vi "correction for PL spectra.vi"(1 "file path (dialog if empty) 2":path caption="PL file needed to be transfromed") -> (0 "数组 2":dbl[][](array[numeric]))   [LabVIEW 2018]
uses:
  <vilib>/Utility/file.llb/Read Delimited Spreadsheet (DBL).vi
panel:
  out "first row":dbl[](array[numeric])
  out "XY Graph":cluster{"Y":dbl[], "Y":dbl[]}[](graph) caption="XY图"
  out "大小":i32
  out "数组":i32[](array[numeric])
  out "all rows 2":dbl[][](array[numeric]) caption="所有行"
  out "all rows":dbl[][](array[numeric]) caption="所有行"
  in  "file path (dialog if empty)":path=path "C:/PLQY corrected 20210803/correction file from 300nm to 1300nm 20230203.dat" caption="correction file from 300nm to 1300nm"
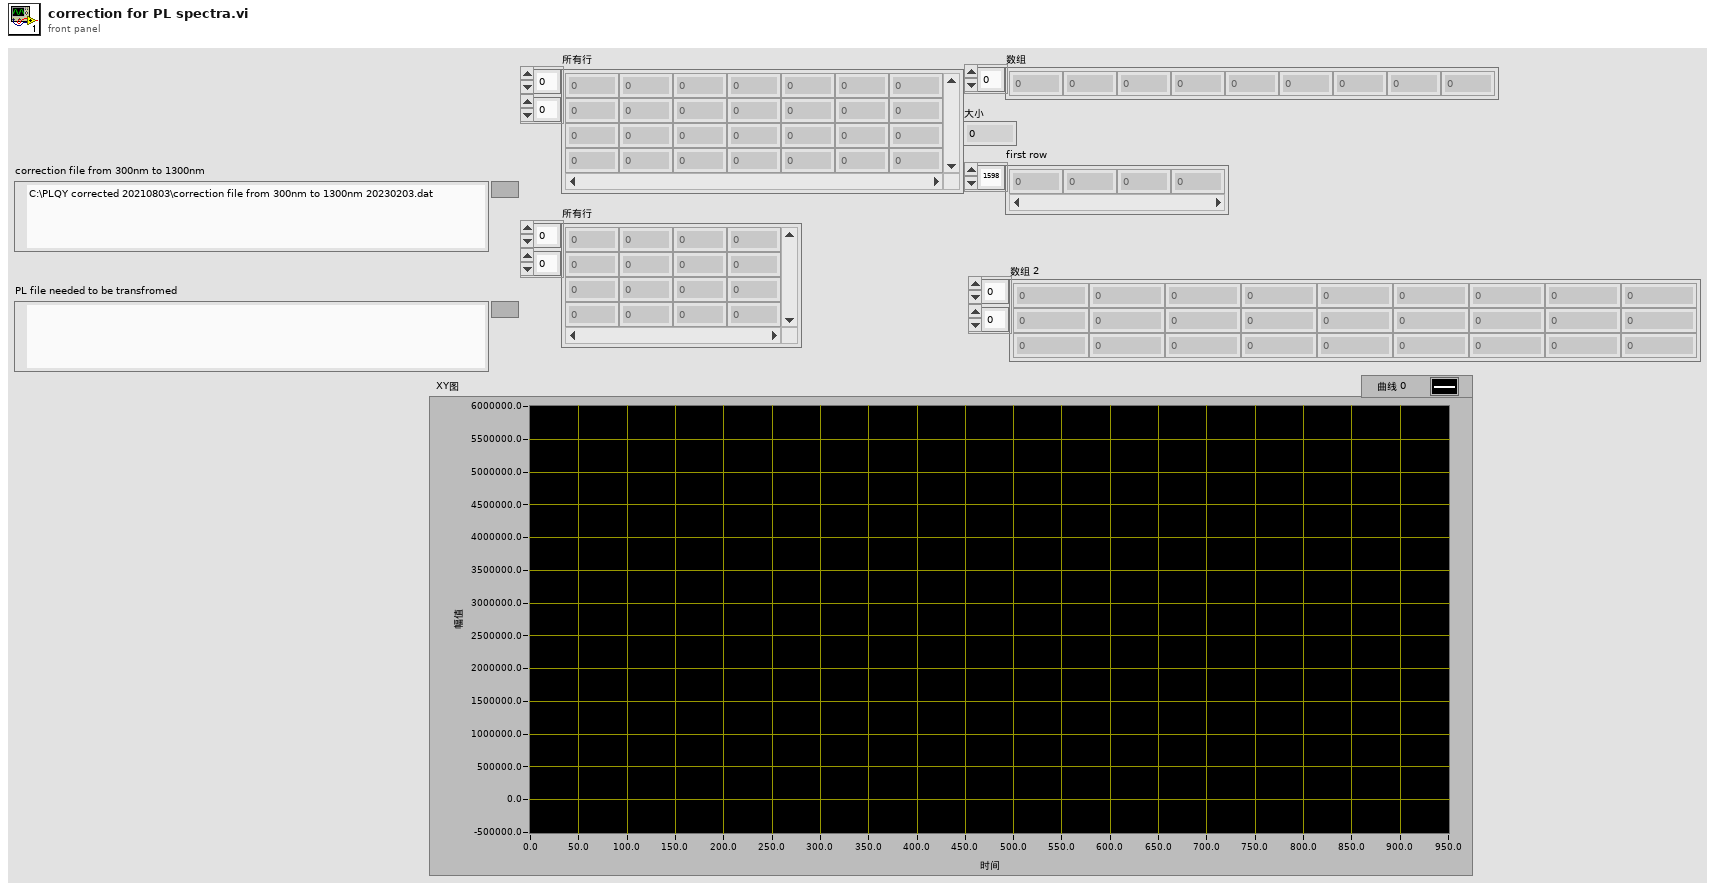
[diagram p1: front panel]
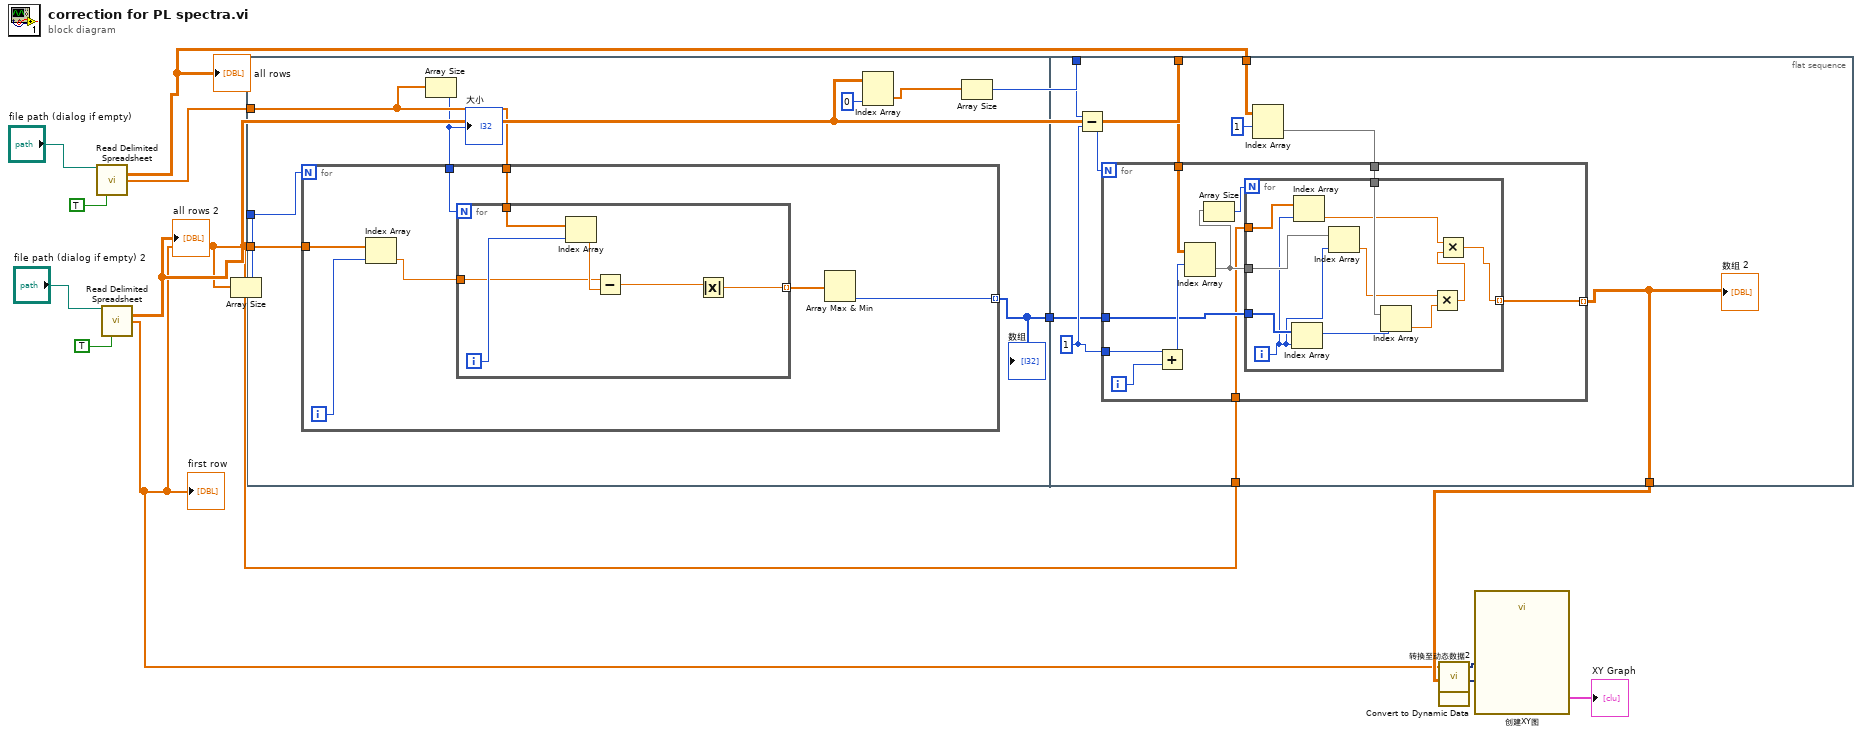
[diagram p0: block diagram]
diagram:
  n1 = call-poly <vilib>:"Read Delimited Spreadsheet.vi"("file path (dialog if empty)"="file path (dialog if empty)", "transpose? (F)"=TRUE) -> ("all rows"=w6:dbl[][], "first row"=w12:dbl[])  [unwired: 8 in, 4 out]
  "all rows" <- w6
  n2 = call-poly <vilib>:"Read Delimited Spreadsheet.vi"("file path (dialog if empty)"="file path (dialog if empty) 2", "transpose? (F)"=TRUE) -> ("all rows"=w11:dbl[][], "first row"=w1:dbl[])  [unwired: 8 in, 4 out]
  "all rows 2" <- w11
  "first row" <- w1
  n3 = Array Size(array=w1) -> (size(s)=w13:i32)
  n4 = flat-sequence {
    tunnel: w1 -> [w22]
    tunnel: w13 -> [w21]
    tunnel: w12 -> [w20]
    tunnel: [w18] -> w7
    tunnel: w11 -> [w41]
    tunnel: w8 -> [w45]
    tunnel: w7 -> [w42]
    tunnel: w6 -> [w38]
    tunnel: w1 -> [w37]
    tunnel: [w36] -> w3
    frame #0 {
      n5 = Array Size(array=w20) -> (size(s)=w19:i32)
      "大小" <- w19
      n6 = for {
        N: w21 -> [_]
        tunnel: w22 -> [w29]
        tunnel: w20 -> [w27]
        tunnel: w19 -> [w26]
        tunnel: [w23] -> w18 mode=indexing
        i -> [w28]
        n7 = Index Array(array=w29, index=w28) -> (element=w25:dbl)
        n8 = for {
          N: w26 -> [_]
          tunnel: w27 -> [w35]
          tunnel: w25 -> [w32]
          tunnel: [w30] -> w24 mode=indexing
          i -> [w34]
          n9 = Index Array(array=w35, index=w34) -> (element=w33:dbl)
          n10 = Subtract(x=w32, y=w33) -> (x-y=w31:dbl)
          n11 = Absolute Value(x=w31) -> (abs(x)=w30:dbl)
        }
        n12 = Array Max & Min(array=w24) -> (min index (indices)=w23:i32)  [unwired: 3 out]
      }
      "数组" <- w18
    }
    frame #1 {
      w44 = 1 ("x")
      n13 = Subtract(x=w45, y=w44) -> (x-y=w43:i32)
      n14 = Index Array(array=w38, index (row)=1 ("索引 (行)")) -> (element=w39:dbl[])  [unwired: 1 in]
      n15 = for {
        N: w43 -> [_]
        tunnel: w44 -> [w54]
        tunnel: w41 -> [w53]
        tunnel: w42 -> [w51]
        tunnel: w39 -> [w50]
        tunnel: [w49] -> w36 mode=indexing
        tunnel: w37 -> [w46]
        i -> [w55]
        n16 = Add(x=w54, y=w55) -> (x+y=w52:i32)
        n17 = Index Array(array=w53, index (row)=w52) -> (element=w47:dbl[])  [unwired: 1 in]
        n18 = Array Size(array=w47) -> (size(s)=w48:i32)
        n19 = for {
          N: w48 -> [_]
          tunnel: w51 -> [w66]
          tunnel: w47 -> [w65]
          tunnel: w50 -> [w64]
          tunnel: [w60] -> w49 mode=indexing
          tunnel: w46 -> [w57]
          i -> [w58]
          n20 = Index Array(array=w66, index=w58) -> (element=w63:i32)
          n21 = Index Array(array=w57, index=w58) -> (element=w56:dbl)
          n22 = Index Array(array=w65, index=w58) -> (element=w61:dbl)
          n23 = Index Array(array=w64, index=w63) -> (element=w62:dbl)
          n24 = Multiply(x=w61, y=w62) -> (x*y=w59:dbl)
          n25 = Multiply(x=w56, y=w59) -> (x*y=w60:dbl)
        }
      }
      "数组 2" <- w36
    }
  }
  n26 = Index Array(array=w11, index (col)=0 ("禁用的索引 (列)")) -> (element=w9:dbl[])  [unwired: 1 in]
  n27 = Array Size(array=w9) -> (size(s)=w8:i32)
  n28 = call "转换至动态数据2"("Array"=w1) -> ("Dynamic Data Type"=w4:dynamicdata)  [unwired: 3 in]
  n29 = call "Convert to Dynamic Data"("2D Array"=w3) -> ("Dynamic Data Type"=w2:dynamicdata)  [unwired: 3 in]
  n30 = call "创建XY图"("Y Input"=w2, "X Input"=w4) -> ("XY Graph"=→"XY Graph":cluster{"X":dbl[], "Y":dbl[]}[])  [unwired: 8 in, 1 out]
